vi "Process-server-message.vi"(8 "error in (no error)":errorcluster, 9 "Message type":T1, 10 "Message":refnum<class "Message.lvclass">, 11 "ModComm in":T2) -> (0 "error out":errorcluster, 1 "Exit?":bool, 3 "ModComm out":T2)   [LabVIEW 2013, in "Server.lvlib" / "Server.lvclass"]
uses:
  Server.lvclass
  Object-reference.ctl
  Messages/Sources/Message.lvclass
  Server-messages.ctl
  Messages/Sources/Error/Error.lvclass
  Messages/Sources/Error/Error.lvclass/Error.ctl
  Messages/Sources/Start-client/Start-client.lvclass
  Messages/Sources/Start-client/Start-client.lvclass/Start-client.ctl
  Messages/Sources/Get-clients/Get-clients.lvclass
  Messages/Sources/Message.lvclass/Message.ctl
  Messages/Sources/Start-client/Read Module path.vi
  Messages/Sources/Start-client/Read Module type.vi
  Messages/Sources/Read Sender type.vi
  Messages/Sources/Read Sender ID.vi
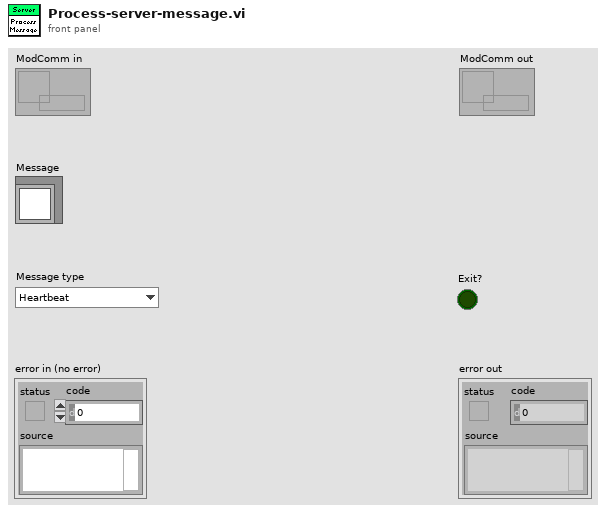
[diagram p1: front panel]
types:
  T1 = typedef "Server.lvlib/Server.lvclass/Server-messages.ctl" = enum16{"Heartbeat", "Error", "Start client", "Client stopped", "Query status", "Send status", "Get clients"}
  T2 = typedef "Server.lvlib/Server.lvclass/Object-reference.ctl" = refnum<data-value>
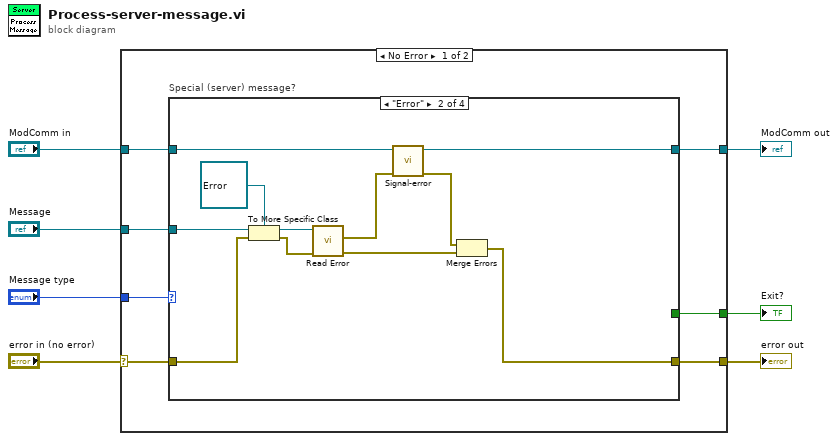
[diagram p0: block diagram]
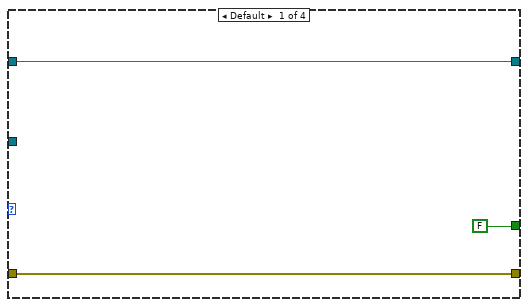
[diagram p2: hidden frame]
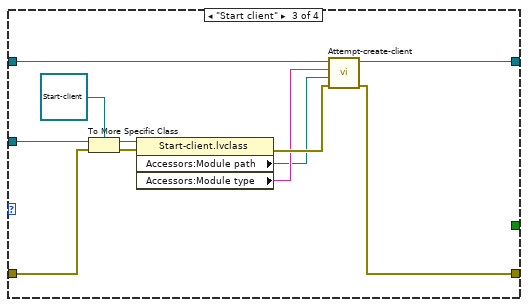
[diagram p3: hidden frame]
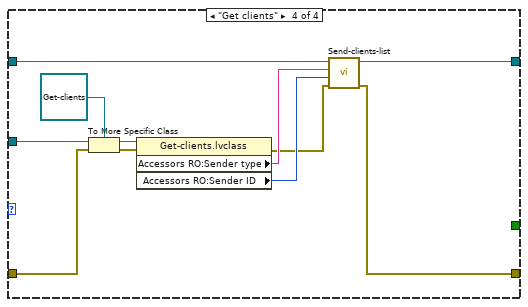
[diagram p4: hidden frame]
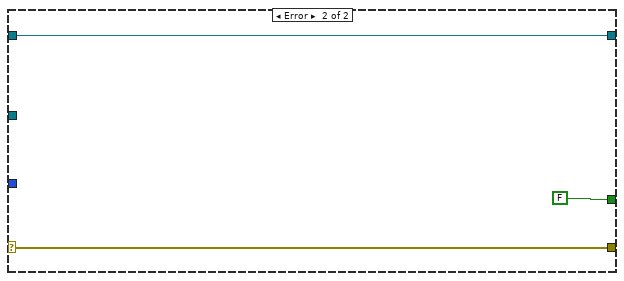
[diagram p5: hidden frame]
diagram:
  n1 = case shown="No Error" "error in (no error)" {
    selector: "error in (no error)" -> [w9 w53]
    tunnel: [w13 w53] -> w6
    tunnel: [w14 w52] -> w4
    tunnel: "ModComm in" -> [w11 w52]
    tunnel: [w8 FALSE] -> w3
    tunnel: "Message" -> [w10 _]
    tunnel: "Message type" -> [w12 _]
    frame No Error {
      n2 = case "Special (server) message?" shown="\"Error\"" w12 {
        tunnel: [w16 w18 w29 w41] -> w13
        tunnel: [w17 w27 w32 w40] -> w14
        tunnel: w11 -> [w17 w28 w34 w43]
        tunnel: w10 -> [_ w26 w39 w50]
        tunnel: w9 -> [w16 w23 w37 w48]
        tunnel: [FALSE _ _ _] -> w8
        frame Default {
        }
        frame "Error" {
          n3 = To More Specific Class(target class=refnum<class "Error.lvclass"> refnum ("Module-communication.lvlib:Error.lvclass"), reference=w26, error in=w23) -> (specific class reference=w24:refnum<class "Error.lvclass">, error out=w22:errorcluster)
          n4 = call "Read Error.vi"("error in (no error)"=w22, "Error in"=w24) -> ("error out"=w19:errorcluster, "Error"=w21:errorcluster)  [unwired: 7 in, 1 out]
          n5 = call "Signal-error.vi"("error in (no error)"=w21, "ModComm in"=w28) -> ("error out"=w20:errorcluster, "ModComm out"=w27:T2)  [unwired: 8 in]
          n6 = Merge Errors(w20, w19) -> (w18:errorcluster)
        }
        frame "Start client" {
          n7 = To More Specific Class(target class=refnum<class "Start-client.lvclass"> refnum ("Module-communication.lvlib:Start-client.lvclass"), reference=w39, error in=w37) -> (specific class reference=w35:refnum<class "Start-client.lvclass">, error out=w36:errorcluster)
          n8 = property class="Start-client.lvclass"(reference=w35, error in=w36) -> (error out=w33:errorcluster, "Accessors:Module path"=w30:path, "Accessors:Module type"=w31:string)  [unwired: 1 out]
          n9 = call "Attempt-create-client.vi"("error in (no error)"=w33, "Module path"=w30, "Module type"=w31, "ModComm in"=w34) -> ("error out"=w29:errorcluster, "ModComm out"=w32:T2)  [unwired: 6 in]
        }
        frame "Get clients" {
          n10 = To More Specific Class(target class=refnum<class "Get-clients.lvclass"> refnum ("Module-communication.lvlib:Get-clients.lvclass"), reference=w50, error in=w48) -> (specific class reference=w46:refnum<class "Get-clients.lvclass">, error out=w47:errorcluster)
          n11 = property class="Get-clients.lvclass"(reference=w46, error in=w47) -> (error out=w42:errorcluster, "Accessors RO:Sender type"=w45:string, "Accessors RO:Sender ID"=w44:i32)  [unwired: 1 out]
          n12 = call "Send-clients-list.vi"("error in (no error)"=w42, "Sender ID"=w44, "Sender"=w45, "ModComm in"=w43) -> ("error out"=w41:errorcluster, "ModComm out"=w40:T2)  [unwired: 6 in]
        }
      }
    }
    frame Error {
    }
  }
  "error out" <- w6
  "ModComm out" <- w4
  "Exit?" <- w3
